vi "Rotation2D_Subtract.vi"(9 "Other ROTATION":T1={"VALUE"=0.0, "COS"=1.0, "SIN"=0.0} {"SIN" format="%13.4f"; "COS" format="%13.4f"; "VALUE" format="%13.4f"}, 11 "In ROTATION":T1={"VALUE"=0.0, "COS"=1.0, "SIN"=0.0} {"SIN" format="%13.4f"; "COS" format="%13.4f"; "VALUE" format="%13.4f"}) -> (3 "Out ROTATION Out":T1 {"SIN" format="%13.4f"; "COS" format="%13.4f"; "VALUE" format="%13.4f"})   [LabVIEW 2020, in "Swerve_Odometry_SEN.lvlib"]
doc: "Subtracts the new rotation from the current rotation and returns the new rotation.\n\nFor example, Rotation2d.fromDegrees(10) - Rotation2d.fromDegrees(100) = Rotation2d{-pi/2}\n\nParameters:\n- in ROTATION - This rotation data structure\n - other ROTATION - The rotation to subtract.\n\nReturns:\n - out ROTATION - The difference between the two rotations."
uses:
  Swerve_Odometry_SEN.lvlib
  Cluster_ROTATION2D.ctl
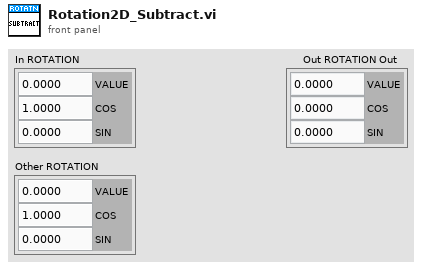
[diagram p1: front panel]
types:
  T1 = typedef "Swerve_Odometry_SEN.lvlib/Cluster_ROTATION2D.ctl" = cluster{"VALUE":dbl, "COS":dbl, "SIN":dbl}
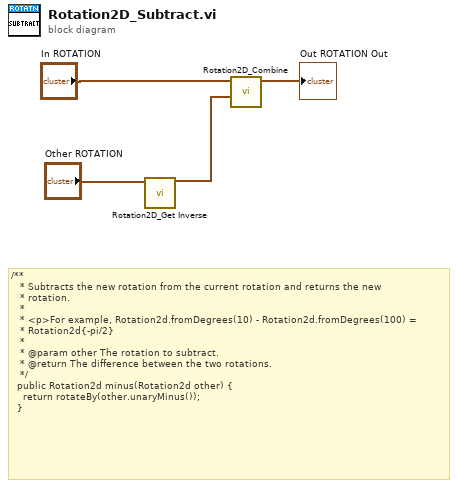
[diagram p0: block diagram]
diagram:
  # "/**\n   * Subtracts the new rotation from the current rotation and returns the new\n   * rotation.\n   *\n   * <p>For example, Rotation2d.fromDegrees(10) - Rotation2d.fromDegrees(100) =\n   * Rotation2d{-pi/2}\n   *\n   * @param other The rotation to subtract.\n   * @return The difference between the two rotations.\n   */\n  public Rotation2d minus(Rotation2d other) {\n    return rotateBy(other.unaryMinus());\n  }"
  n1 = call "Rotation2D_Get Inverse.vi"("ROTATION"="Other ROTATION") -> ("Inverse ROTATION"=w2:T1)  [unwired: 10 in]
  n2 = call "Rotation2D_Combine.vi"("other Rotation"=w2, "in ROTATION"="In ROTATION") -> ("out ROTATION"=→"Out ROTATION Out":T1)  [unwired: 9 in]
